vi "Result All Steps Judgement Codes.vi"(8 "error in (no error)":errorcluster, 11 "VISA resource name":refnum<visa-resource-name>) -> (0 "error out":errorcluster, 2 "Results":string, 3 "VISA resource name out":refnum<visa-resource-name>)   [LabVIEW 2025, in "Chroma 19052.lvlib"]
uses:
  <instrlib>/Chroma 19052/Chroma 19052.lvlib
  <vilib>/Utility/error.llb/Trim Whitespace One-Sided.vi
panel:
  # "All Steps Judgement Codes Results query"
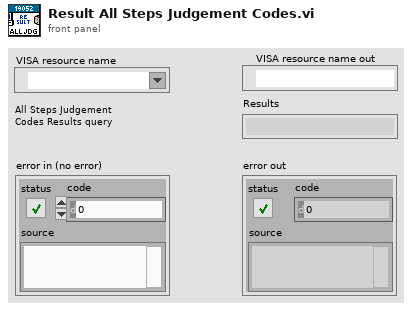
[diagram p1: front panel]
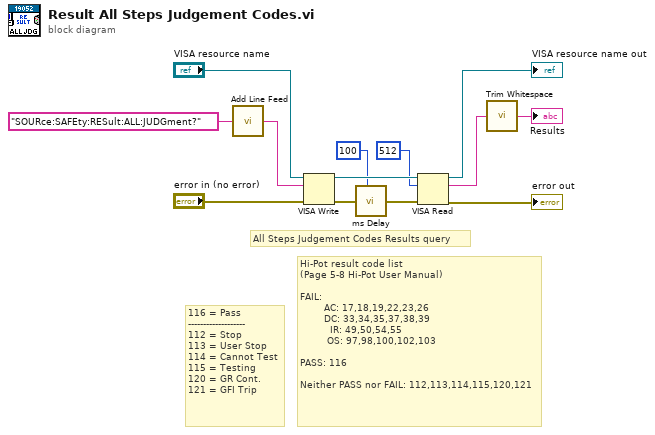
[diagram p0: block diagram]
diagram:
  # "Hi-Pot result code list \n(Page 5-8 Hi-Pot User Manual)\n\nFAIL: \n        AC: 17,18,19,22,23,26\n        DC: 33,34,35,37,38,39\n          IR: 49,50,54,55\n         OS: 97,98,100,102,103\n\nPASS: 116\n\nNeither PASS nor FAIL: 112,113,114,115,120,121"
  # "116 = Pass\n-------------------\n112 = Stop\n113 = User Stop\n114 = Cannot Test\n115 = Testing\n120 = GR Cont.\n121 = GFI Trip"
  # "All Steps Judgement Codes Results query"
  n1 = call <instrlib>:"Add Line Feed.vi"("Command string"="SOURce:SAFEty:RESult:ALL:JUDGment?") -> ("Concatenated string"=w2:string)  [unwired: 4 in]
  n2 = VISA Write(VISA resource name="VISA resource name", write buffer=w2, error in (no error)="error in (no error)") -> (VISA resource name out=w13:refnum<visa-resource-name>, error out=w8:errorcluster)  [unwired: 1 out]
  n3 = call <instrlib>:"ms Delay.vi"("miliseconds to wait"=u32 100, "error in (no error)"=w8) -> ("error out"=w7:errorcluster)  [unwired: 6 in, 1 out]
  n4 = VISA Read(VISA resource name=w13, byte count=u32 512, error in (no error)=w7) -> (VISA resource name out=→"VISA resource name out":refnum<visa-resource-name>, read buffer=w9:string, error out=→"error out":errorcluster)  [unwired: 1 out]
  n5 = call <vilib>:"Trim Whitespace.vi"("string"=w9) -> ("trimmed string"=→"Results":string)  [unwired: 1 in]
